vi "Largest Buffer Size (Transfer Group).vi"(8 "error in (no error)":errorcluster, 9 "prev engine buffer size (0)":u64 format="%d bytes", 10 "prev string buffer size (0)":u64 format="%d bytes", 11 "Transfer Group Configuration in":T1={"core"={"name"="", "direction"=enum."Rx", "cycle timing"={"priority"=0, "decimation"=0, "offset"=255}, "timeout behavior"=enum."Increment Late Count"}, "component settings"=[], "transfers"=[]} {"transfers"."channels"."core"."string offset" format="%d bytes"}) -> (0 "error out":errorcluster, 1 "largest engine buffer size":u64 format="%d bytes", 2 "largest string buffer size":u64 format="%d bytes", 3 "Transfer Group Configuration out":T1={"core"={"name"="", "direction"=enum."Rx", "cycle timing"={"priority"=0, "decimation"=0, "offset"=255}, "timeout behavior"=enum."Increment Late Count"}, "component settings"=[], "transfers"=[]} {"transfers"."channels"."core"."string offset" format="%d bytes"})   [LabVIEW 2017, in "DSF Core.lvlib" / "Configuration Session.lvclass"]
uses:
  Configuration Session.lvclass
  Typedefs/DSF Engine Transfer Group Configuration.ctl
  Typedefs/DSF Core Group Configuration.ctl
  Typedefs/DSF Direction.ctl
  Typedefs/DSF Timing Info.ctl
  Typedefs/DSF Timeout Behavior.ctl
  Typedefs/DSF Settings Info.ctl
  Typedefs/DSF Version Info.ctl
  Typedefs/DSF Engine Transfer Configuration.ctl
  Typedefs/DSF Core Transfer Configuration.ctl
  Typedefs/DSF Engine Channel Configuration.ctl
  Typedefs/DSF Core Channel Configuration.ctl
  Typedefs/DSF Data Type.ctl
  DSF Core.lvlib
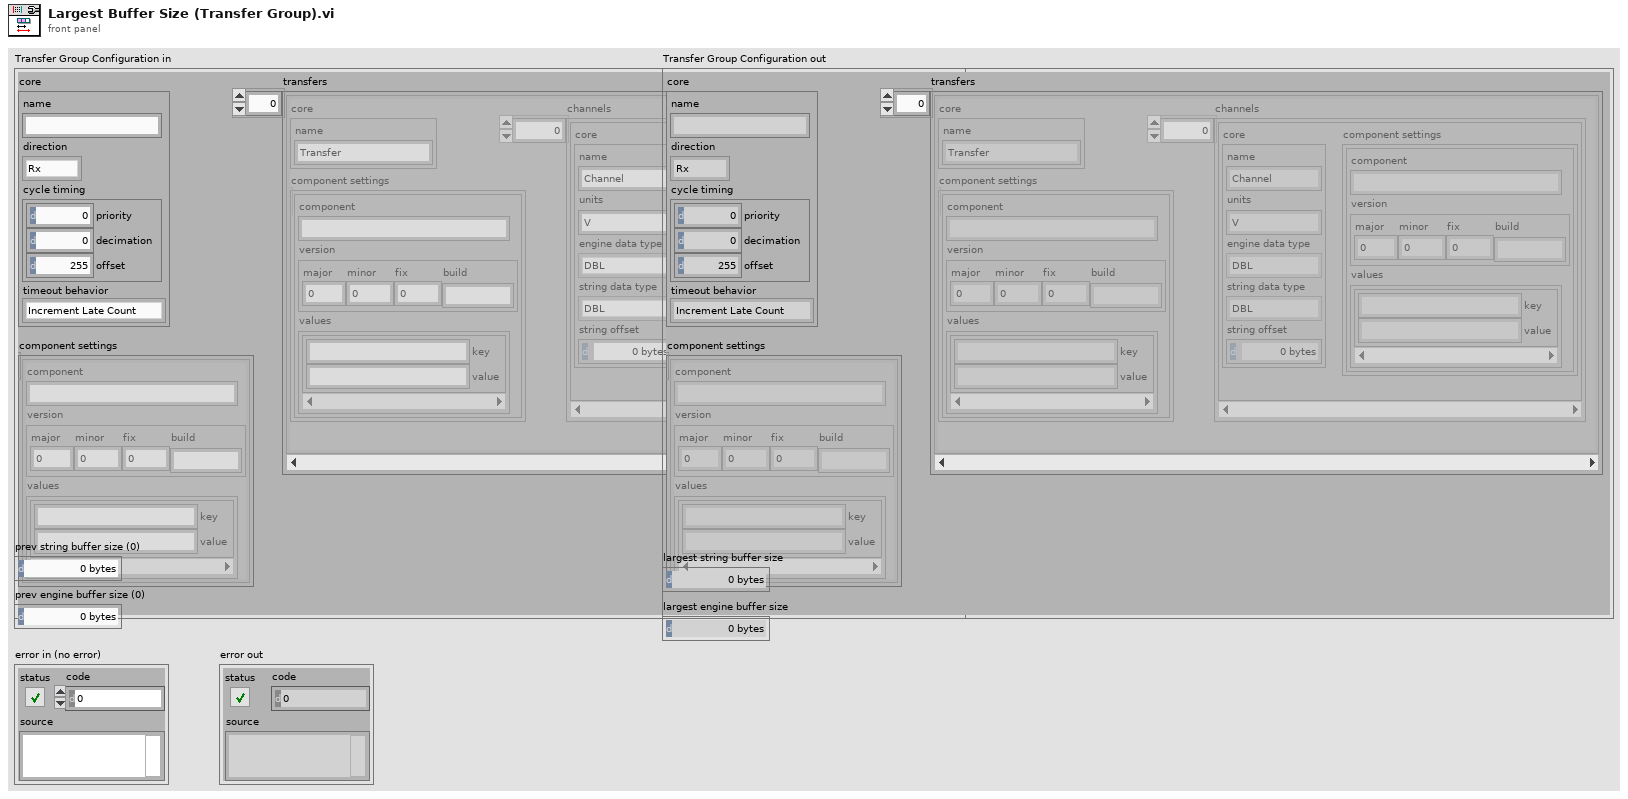
[diagram p1: front panel]
types:
  T1 = typedef "DSF Core.lvlib/DSF Engine Transfer Group Configuration.ctl" = cluster{"core":T2, "component settings":T6[], "transfers":T8[]}
  T2 = typedef "DSF Core.lvlib/DSF Core Group Configuration.ctl" = cluster{"name":string, "direction":T3, "cycle timing":T4, "timeout behavior":T5}
  T3 = typedef "DSF Core.lvlib/DSF Direction.ctl" = enum8{"Tx", "Rx"}
  T4 = typedef "DSF Core.lvlib/DSF Timing Info.ctl" = cluster{"priority":u64, "decimation":u64, "offset":u64}
  T5 = typedef "DSF Core.lvlib/DSF Timeout Behavior.ctl" = enum8{"Increment Late Count", "Throw Error"}
  T6 = typedef "DSF Core.lvlib/DSF Settings Info.ctl" = cluster{"component":string, "version":T7, "values":cluster{"key":string, "value":string}[]}
  T7 = typedef "DSF Core.lvlib/DSF Version Info.ctl" = cluster{"major":u32, "minor":u32, "fix":u32, "build":string}
  T8 = typedef "DSF Core.lvlib/DSF Engine Transfer Configuration.ctl" = cluster{"core":T9, "component settings":T6[], "channels":T10[]}
  T9 = typedef "DSF Core.lvlib/DSF Core Transfer Configuration.ctl" = cluster{"name":string}
  T10 = typedef "DSF Core.lvlib/DSF Engine Channel Configuration.ctl" = cluster{"core":T11, "component settings":T6[]}
  T11 = typedef "DSF Core.lvlib/DSF Core Channel Configuration.ctl" = cluster{"name":string, "units":string, "engine data type":T12, "string data type":T12, "string offset":u64}
  T12 = typedef "DSF Core.lvlib/DSF Data Type.ctl" = enum8{"Bool", "SGL", "DBL", "I8", "I16", "I32", "I64", "U8", "U16", "U32", "U64"}
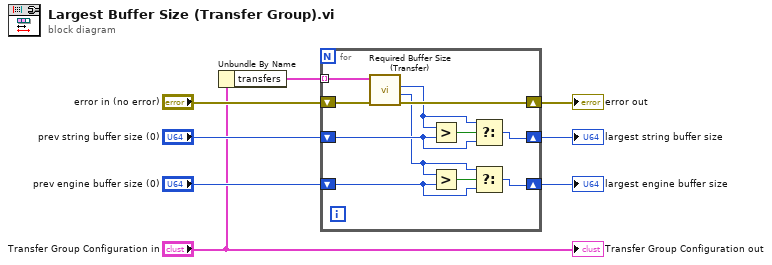
[diagram p0: block diagram]
diagram:
  n1 = Unbundle By Name("Transfer Group Configuration in") -> ("transfers"=w7:T8[])
  n2 = for {
    tunnel: w7 -> [w19] mode=indexing
    shift-right: [w15] -> w8
    shift-left: "prev string buffer size (0)" -> [w14]
    shift-right: [w18] -> w5
    shift-left: "error in (no error)" -> [w17]
    shift-right: [w9] -> w4
    shift-left: "prev engine buffer size (0)" -> [w11]
    n3 = call "Required Buffer Size (Transfer).vi"("error in (no error)"=w17, "Transfer Configuration in"=w19) -> ("error out"=w18:errorcluster, "engine buffer size"=w10:u64, "string buffer size"=w13:u64)  [unwired: 6 in, 1 out]
    n4 = Greater?(x=w13, y=w14) -> (0:w16:bool)
    n5 = Greater?(x=w10, y=w11) -> (0:w12:bool)
    n6 = Select(t=w13, s=w16, f=w14) -> (s? t:f=w15:u64)
    n7 = Select(t=w10, s=w12, f=w11) -> (s? t:f=w9:u64)
  }
  "largest string buffer size" <- w8
  "error out" <- w5
  "largest engine buffer size" <- w4
  "Transfer Group Configuration out" <- "Transfer Group Configuration in"
